vi "SkipMusicCommand_Create.vi"(0 "reference in":refnum<class "SkipMusicCommand.lvclass">, 11 "Error In":errorcluster) -> (4 "reference out":refnum<class "SkipMusicCommand.lvclass">, 15 "Error Out":errorcluster)   [LabVIEW 2024, in "SkipMusicCommand.lvclass"]
uses:
  SkipMusicCommand.lvclass/SkipMusicCommand.ctl
  SkipMusicCommand.lvclass
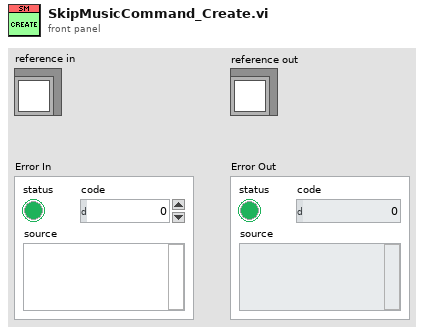
[diagram p1: front panel]
types:
  T1 = typedef "SkipMusicCommand.lvclass/ObjectAttributes.ctl" = cluster{"MediaPlayerRef":refnum<class "MediaPlayer.lvclass">}
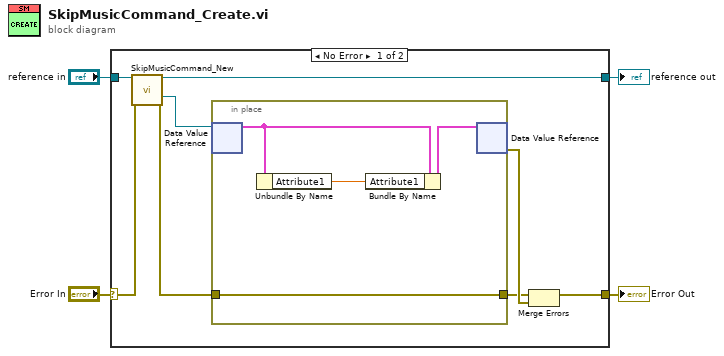
[diagram p0: block diagram]
diagram:
  n1 = case shown="No Error" "Error In" {
    selector: "Error In" -> [w11 w18]
    tunnel: [w5 w18] -> w3
    tunnel: "reference in" -> [w12 w17]
    tunnel: [w10 w17] -> w1
    frame No Error {
      n2 = call "SkipMusicCommand_New.vi"("reference in"=w12, "Error In"=w11) -> ("reference out"=w10:refnum<class "SkipMusicCommand.lvclass">, "DVRRefOut"=w8:refnum<data-value>, "Error Out"=w7:errorcluster)  [unwired: 10 in, 1 out]
      n3 = in-place {
        in-place-border: w7 -> [w13]
        in-place-border: [w13] -> w6
        n4 = in-place-dvr #1(w8) -> (w15:T1)  [unwired: 1 out]
        n5 = Unbundle By Name(w15) -> ("Attribute1"=w14:dbl)
        n6 = Bundle By Name(cluster=w15, "Attribute1"=w14) -> (w16:T1)
        n7 = in-place-dvr #1(w16) -> (w9:errorcluster)  [unwired: 1 out]
      }
      n8 = Merge Errors(w6, w9) -> (w5:errorcluster)
    }
    frame Error {
      # "VI-TechBaseTemplate_Simple_4x4x4"
    }
  }
  "Error Out" <- w3
  "reference out" <- w1
